vi "LVFunction_Imop_SlopesCompute_ModalCoef.vi"(0 "ModalCoef":refnum<class "ModalCoef.lvclass">, 1 "ComputePhaseSet":refnum<class "ComputePhaseSet.lvclass">, 2 "HasoSlopes":refnum<class "HasoSlopes.lvclass">) -> (4 "ModalCoef (dup)":refnum<class "ModalCoef.lvclass">)   [LabVIEW 2020]
doc: "Compute modal coefficients that represent slopes in a given basis of\npolynomials provided by ComputePhaseSet.\n\n--------------------------------------------------------------------------------\n\nHasoDataIn\n HasoData object.\n\nHasoDataOut\n HasoData object.\n\nComputePhaseSet\n cComputePhaseSet object.\n\nmodalCoef\n cModalCoef object.\n\nErrorIn\n Error\nErrorOut\n Error"
uses:
  ComputePhaseSet.lvclass
  ModalCoef.lvclass
  HasoSlopes.lvclass
  LVClass_ModalCoef Read ModalCoef.vi
  LVClass_ComputePhaseSet Read ComputePhaseSet.vi
  LVClass_HasoSlopes Read HasoSlopes _ property.vi
panel:
  out "error out":errorcluster
  in  "error constant":errorcluster
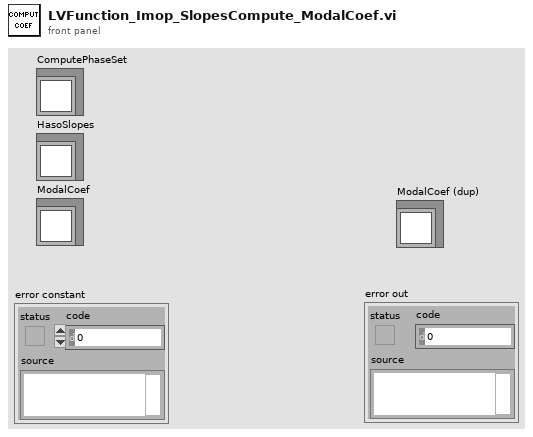
[diagram p1: front panel]
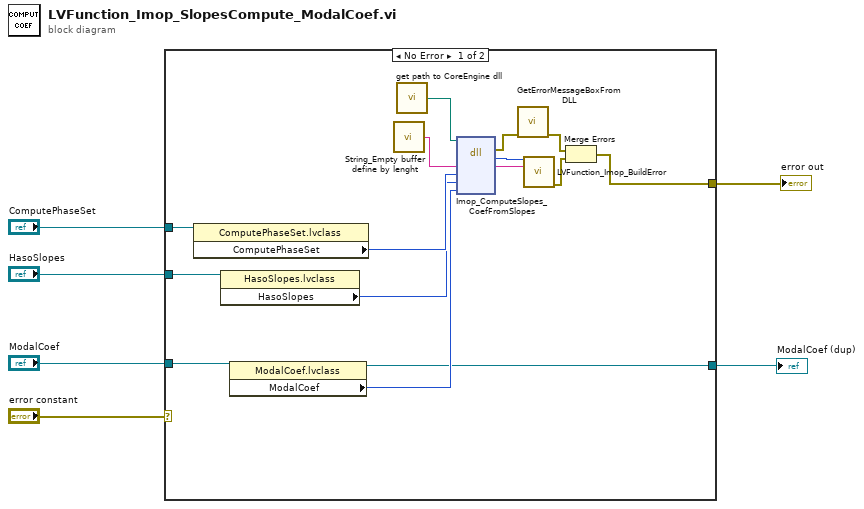
[diagram p0: block diagram]
diagram:
  n1 = case shown="No Error" "error constant" {
    selector: "error constant" -> [_ w23]
    tunnel: "HasoSlopes" -> [w16 _]
    tunnel: "ComputePhaseSet" -> [w15 _]
    tunnel: [w8 w23] -> w5
    tunnel: "ModalCoef" -> [w12 w22]
    tunnel: [w7 w22] -> w2
    frame No Error {
      n2 = property class="ComputePhaseSet.lvclass"(reference=w15) -> ("ComputePhaseSet"=w14:i32)  [unwired: 1 in, 2 out]
      n3 = property class="HasoSlopes.lvclass"(reference=w16) -> ("HasoSlopes"=w13:i32)  [unwired: 1 in, 2 out]
      n4 = property class="ModalCoef.lvclass"(reference=w12) -> (reference out=w7:refnum<class "ModalCoef.lvclass">, "ModalCoef"=w11:u32)  [unwired: 1 in, 1 out]
      n5 = call "String_Empty buffer define by lenght.vi"() -> ("Empty buffer"=w19:string)  [unwired: 1 in]
      n6 = call "get path to CoreEngine dll.vi"() -> ("path to c_interface_vc100.dll"=w18:path)  [unwired: 12 in, 3 out]
      n7 = dll-call lib="D:/FLE/0.Code/CoreEngine4_Suite/LV2011_interface/DLLs/c_interface_vc100.dll" fn="Imop_ComputeSlopes_CoefFromSlopes"(path in=w18, "message"=w19, "ComputePhaseSet"=w14, "HasoSlopes"=w13, "ModalCoeffs"=w11) -> (error out=w17:errorcluster, "return type"=w21:i32, "message"=w20:string)  [unwired: 5 in, 1 out]
      n8 = call "GetErrorMessageBoxFromDLL.vi"("error IN"=w17) -> ("error OUT"=w10:errorcluster)  [unwired: 10 in]
      n9 = call "LVFunction_Imop_BuildError.vi"("code"=w21, "String to Prepend to source (\"\")"=w20) -> ("error out"=w9:errorcluster)  [unwired: 13 in]
      n10 = Merge Errors(w10, w9) -> (w8:errorcluster)
    }
    frame Error {
    }
  }
  "error out" <- w5
  "ModalCoef (dup)" <- w2
